vi "2.5.vi"() -> ()   [LabVIEW 2017]
panel:
  in  "bpm":dbl
  in  "stop":bool
  out "Boolean":bool
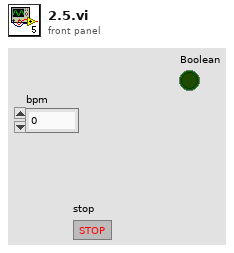
[diagram p1: front panel]
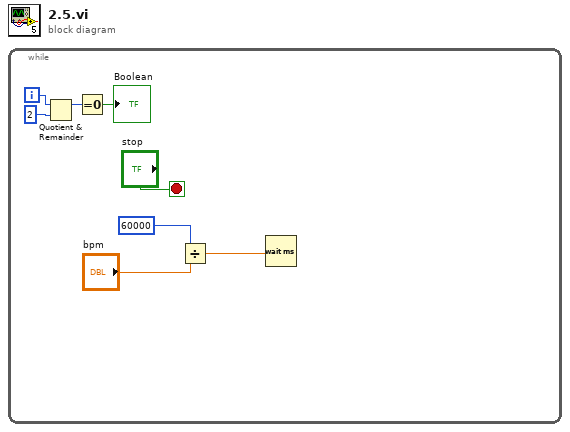
[diagram p0: block diagram]
diagram:
  n1 = while {
    i -> [w8]
    stop <- "stop" stop-if-true
    n2 = Quotient & Remainder(x=w8, y=2) -> (x-y*floor(x/y)=w5:i32)  [unwired: 1 out]
    n3 = Equal To 0?(x=w5) -> (x = 0?=→"Boolean":bool)
    n4 = Divide(x=60000, y="bpm") -> (x/y=w1:dbl)
    n5 = Wait (ms)(milliseconds to wait=w1) -> ()  [unwired: 1 out]
  }
